vi "MQTT_UnsubAck_Read.vi"(8 "error in (no error)":errorcluster, 9 "timeout ms (25000)":i32=25000, 11 "connection ID":refnum<k5>) -> (0 "error out":errorcluster, 2 "MessageID":u16, 3 "connection ID out":refnum<k5>)   [LabVIEW 2018, in "MQTT_Functions.lvlib"]
uses:
  MQTT_Functions.lvlib
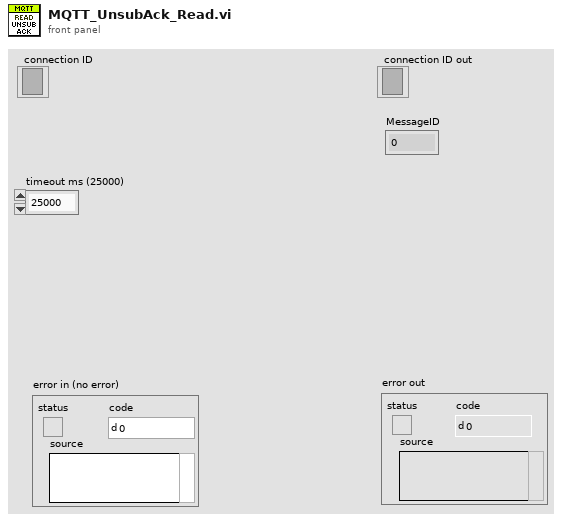
[diagram p1: front panel]
types:
  T1 = typedef "MQTT_Functions.lvlib/MessageType.ctl" = enum32{"Reserved", "CONNECT", "CONNACK", "PUBLISH", "PUBACK", "PUBREC", "PUBREL", "PUBCOMP", "SUBSCRIBE", "SUBACK", "UNSUBSCRIBE", "UNSUBACK", "PINGREQ", "PINGRESP", "DISCONNECT", "Reserved2"}
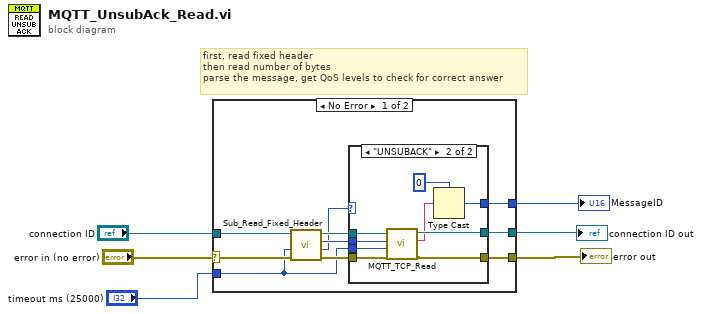
[diagram p0: block diagram]
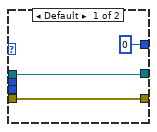
[diagram p2: hidden frame]
diagram:
  # "first, read fixed header\nthen read number of bytes\nparse the message, get QoS levels to check for correct answer"
  n1 = case shown="No Error" "error in (no error)" {
    selector: "error in (no error)" -> [w13 w30]
    tunnel: [w12 w30] -> w5
    tunnel: "timeout ms (25000)" -> [w11 _]
    tunnel: "connection ID" -> [w10 w29]
    tunnel: [w9 w29] -> w2
    tunnel: [w8 _] -> w1
    frame No Error {
      n2 = call "Sub_Read_Fixed_Header.vi"("error in (no error)"=w13, "timeout ms (25000)"=w11, "connection ID"=w10) -> ("error out"=w15:errorcluster, "MessageType"=w7:T1, "Remaining Length"=w16:u32, "connection ID out"=w14:refnum<k5>)  [unwired: 2 in, 3 out]
      n3 = case shown="\"UNSUBACK\"" w7 {
        tunnel: w16 -> [_ w28]
        tunnel: w15 -> [w17 w27]
        tunnel: w14 -> [w18 w26]
        tunnel: [w17 w25] -> w12
        tunnel: w11 -> [_ w24]
        tunnel: [w18 w23] -> w9
        tunnel: [u16 0 w20] -> w8
        frame Default {
        }
        frame "UNSUBACK" {
          n4 = call "MQTT_TCP_Read.vi"("error in (no error)"=w27, "timeout ms (25000)"=w24, "bytes to read"=w28, "connection ID"=w26) -> ("error out"=w25:errorcluster, "data out"=w22:string, "connection ID out"=w23:refnum<k5>)  [unwired: 5 in]
          n5 = Type Cast(type=u16 0, x=w22) -> (*(type *) &x=w20:u16)
        }
      }
    }
    frame Error {
    }
  }
  "error out" <- w5
  "connection ID out" <- w2
  "MessageID" <- w1
